vi "Read Time.vi"(8 "error in (no error)":errorcluster, 11 "ControlMouseEnterMsg in":refnum<class "ControlMouseEnterMsg.lvclass">) -> (0 "error out":errorcluster, 2 "Time":u32, 3 "ControlMouseEnterMsg out":refnum<class "ControlMouseEnterMsg.lvclass">)   [LabVIEW 2018, in "MVA Framework.lvlib" / "ActorEvents.lvlib" / "ControlMouseEnterMsg.lvclass"]
uses:
  ControlMouseEnterMsg.lvclass
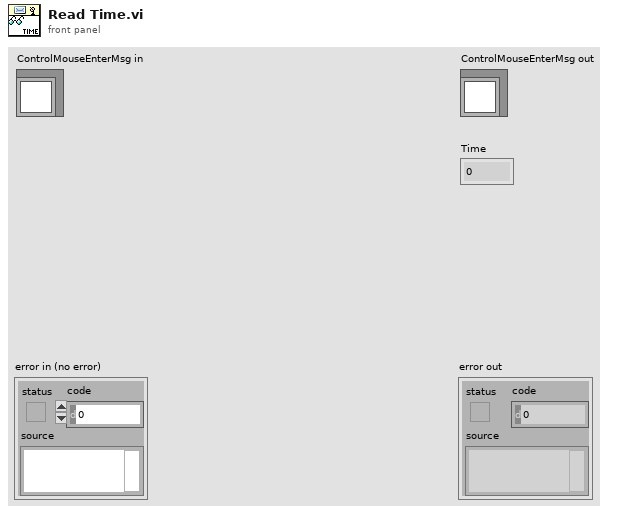
[diagram p1: front panel]
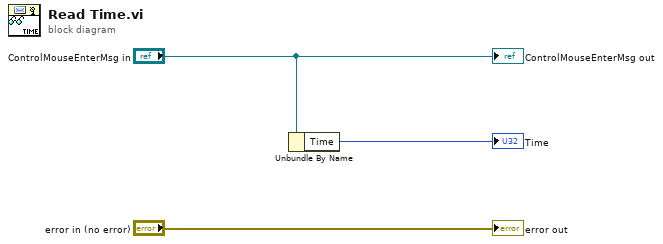
[diagram p0: block diagram]
diagram:
  n1 = Unbundle By Name("ControlMouseEnterMsg in") -> ("Time"=→"Time":u32)
  "error out" <- "error in (no error)"
  "ControlMouseEnterMsg out" <- "ControlMouseEnterMsg in"
